vi "Move Motor Relative.vi"(7 "Mono System # (0)":T1, 8 "error in (no error)":errorcluster, 10 "Steps to Move":dbl, 11 "VISA resource name":refnum<visa-resource-name>) -> (0 "error out":errorcluster, 3 "VISA resource name out":refnum<visa-resource-name>)   [LabVIEW 2009, in "JY-SPEX-TRIAX.lvlib"]
doc: "Moves the spectrometer's motor a relative number of steps from its current position. The motor starts at the minimum speed and ramps up to the maximum (using parameters set by <B>Set Motor Speed.vi</B>). Returns control immediately (before the slits are done moving).\n\nOnly one stepper motor can move at a time; thus, this command cannot be issued if either the slits or the wavelength drive are being moved. Test the motor busy status (using <B>Check Motor Busy.vi</B>) and wait until no motors are busy.\n\nA positive number of steps moves the spectral position forward (greater step position), while a negative number of steps does the reverse. Note that this command does not correct for backlash; that must be done manually.\n\nThe limit to the number of steps that can be moved is the total number of possible steps for the spectrometer."
uses:
  JY-SPEX-TRIAX.lvlib
  controls.llb/Monochromator System Number.ctl
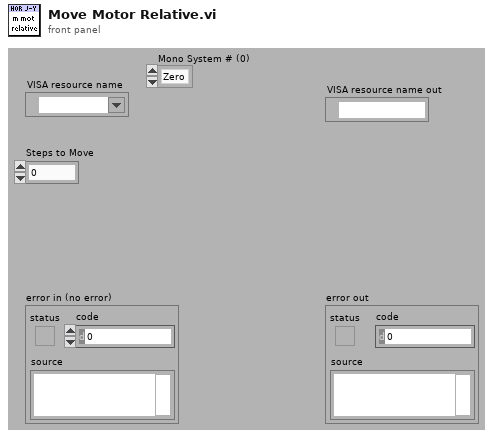
[diagram p1: front panel]
types:
  T1 = typedef "JY-SPEX-TRIAX.lvlib/Monochromator System Number.ctl" = enum16{"Zero", "One"}
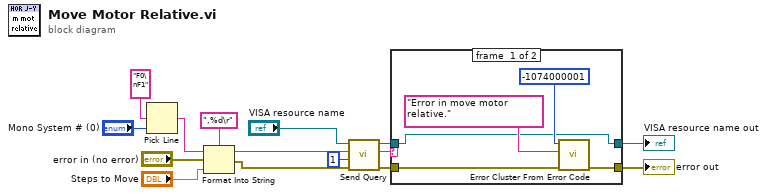
[diagram p0: block diagram]
diagram:
  n1 = Pick Line(multi-line string="F0\nF1", line index="Mono System # (0)") -> (output string=w13:string)  [unwired: 1 out]
  n2 = Format Into String(format string=",%d\r", initial string=w13, error in="error in (no error)", "Steps to Move") -> (resulting string=w11:string, error out=w8:errorcluster)
  n3 = call "Send Query.vi"("error in (no error)"=w8, "byte count"=u32 1, "write buffer"=w11, "VISA resource name"="VISA resource name") -> ("error out"=w3:errorcluster, "read buffer"=w6:string, "VISA resource name out"=w5:refnum<visa-resource-name>)  [unwired: 5 out]
  n4 = case shown="Default" w6 {
    tunnel: w5 -> [w16 w22]
    tunnel: [w16 w22] -> w4
    tunnel: w3 -> [w18 w21]
    tunnel: [w17 w21] -> w2
    frame #0 {
      n5 = call <vilib>:"Error Cluster From Error Code.vi"("error in (no error)"=w18, "error message (\"\")"="Error in move motor relative." ("error message (\"\")"), "error code (0)"=-1074000001) -> ("error out"=w17:errorcluster)  [unwired: 1 in, 5 out]
    }
    frame #1 {
    }
  }
  "VISA resource name out" <- w4
  "error out" <- w2
